vi "SolveSudoku_Labview.vi"() -> ()   [LabVIEW 2023]
uses:
  <vilib>/picture/picture.llb/imagedata.ctl
  <vilib>/Utility/error.llb/Error Cluster From Error Code.vi
  <vilib>/ErrorRing/Error Ring.xnode
panel:
  in  "oPENpdf":bool
  out "subset rect out":T1
  out "Analyse des pixels":bool[][](array[boolean])
  out "resulting number":string
  in  "appel du matlab":bool
  out "Gestion des erreurs":errorcluster
  out "standard error":string
  out "standard output":string
  out "Rectangle.bottom":i16
  out "Rectangle.right":i16
  out "image data":T2
  out "case analysée par le C":picture
  out "Sudoku en entrée":picture
  in  "path to JPEG file":path
  # "SUDOKU SOLVER  :  VEUILLIEZ INSERER UNE GRILLE DE SUDOKU NON RESOLUE DANS LE PORTE DOCUMENT JAUNE ET  LE PROGRAMME VOUS RENVERRA LE SUDOKU RESOLUE !!!\n                     (si vous rentrer une grille qui n'est pas solvable ou avec des dimensions qui ne sont pas normées, le programme vous renverra une erreur ou un warning)"
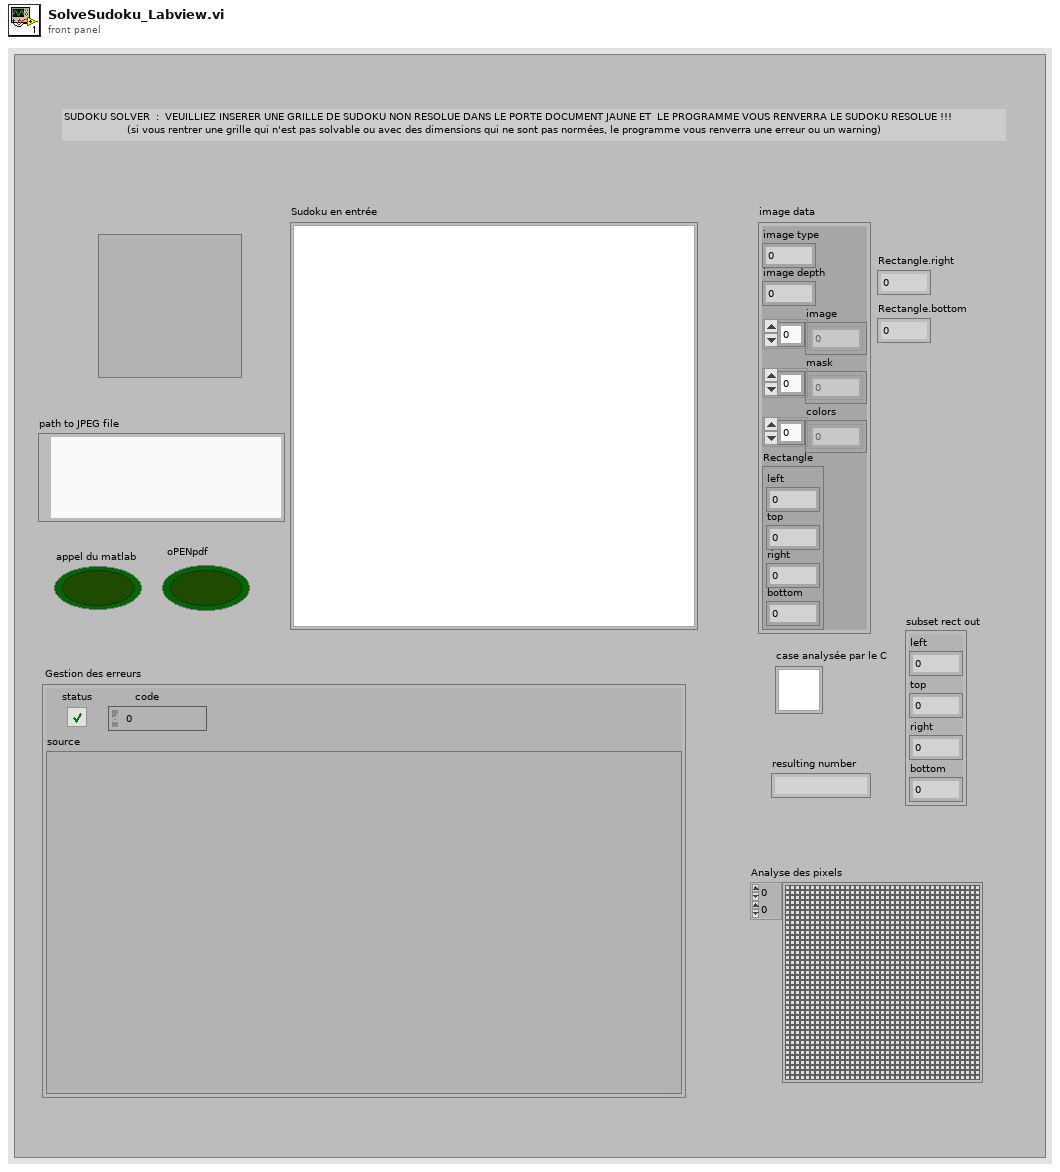
[diagram p1: front panel]
types:
  T1 = cluster{"left":i16, "top":i16, "right":i16, "bottom":i16}
  T2 = typedef "imagedata.ctl" = cluster{"image type":i32, "image depth":i32, "image":u8[], "mask":u8[], "colors":u32[], "Rectangle":cluster{"left":i16, "top":i16, "right":i16, "bottom":i16}}
  T3 = enum16{"open", "replace", "create", "open or create", "replace or create", "replace or create with confirmation"}
  T4 = enum16{"big-endian, network order", "native, host order", "little-endian"}
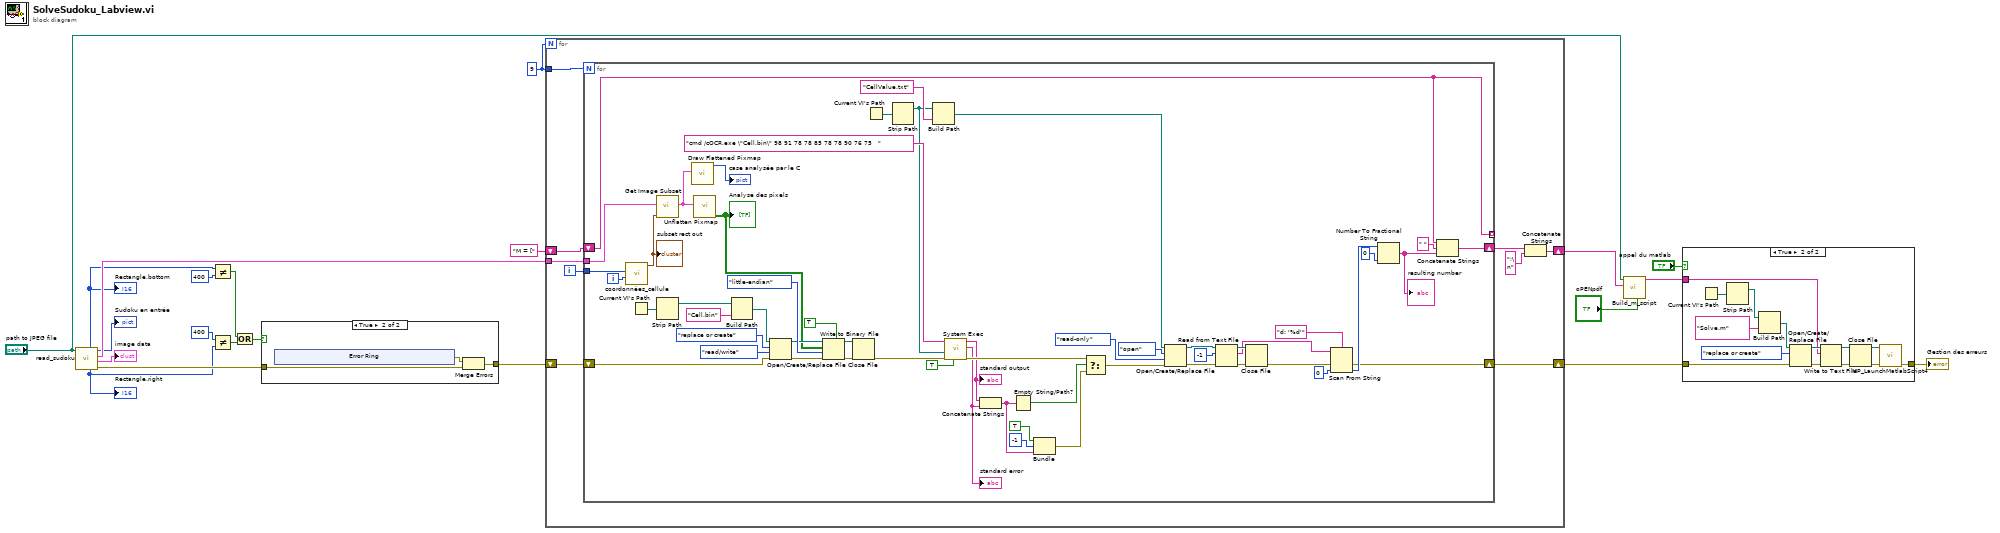
[diagram p0: block diagram]
diagram:
  w21 = 9
  n1 = call "read_sudoku.vi"("path to JPEG file"="path to JPEG file") -> ("gestion des erreurs"=w9:errorcluster, "image data"=→"image data":T2, "image data 2"=w12:T2, "new picture"=→"Sudoku en entrée":picture, "Rectangle.right"=w7:i16, "Rectangle.bottom"=w5:i16)  [unwired: 5 in]
  "Rectangle.right" <- w7
  "Rectangle.bottom" <- w5
  n2 = Not Equal?(x=w5, y=400) -> (x != y?=w3:bool)
  n3 = Not Equal?(x=400, y=w7) -> (x != y?=w2:bool)
  n4 = Or(x=w3, y=w2) -> (x .or. y?=w1:bool)
  n5 = case shown="True" w1 {
    tunnel: [w22 w23] -> w8
    tunnel: w9 -> [w22 w24]
    frame False {
    }
    frame True {
      n6 = xnode "Error Ring"() -> ("error out"=w25:errorcluster)
      n7 = Merge Errors(w25, w24) -> (w23:errorcluster)
    }
  }
  n8 = for {
    N: w21 -> [_]
    tunnel: w12 -> [w39]
    tunnel: w21 -> [w38]
    shift-right: [w34] -> w16
    shift-left: "M = [" ("String") -> [w33]
    shift-right: [w32] -> w19
    shift-left: w8 -> [w31]
    i -> [w37]
    n9 = for {
      N: w38 -> [_]
      tunnel: w39 -> [w91]
      tunnel: w37 -> [w53]
      shift-right: [w67] -> w36
      shift-left: w33 -> [w66]
      tunnel: [w66] -> _ mode=indexing
      shift-right: [w55] -> w32
      shift-left: w31 -> [w64]
      i -> [w52]
      n10 = call "coordonnées_cellule.vi"("Numeric"=w52, "Numeric 2"=w53) -> ("subset rect out"=w51:T1)  [unwired: 9 in]
      "subset rect out" <- w51
      n11 = Current VI's Path() -> (path=w78:path)
      n12 = call <vilib>:"Get Image Subset.vi"("subset rect"=w51, "image data"=w91) -> ("image subset"=w92:T2)  [unwired: 4 in, 1 out]
      n13 = Strip Path(path=w78) -> (stripped path=w90:path)  [unwired: 1 out]
      n14 = call <vilib>:"Draw Flattened Pixmap.vi"("image data"=w92) -> ("new picture"=→"case analysée par le C":picture)  [unwired: 8 in]
      n15 = call <vilib>:"Unflatten Pixmap.vi"("image data"=w92) -> ("1-bit pixmap"=w56:bool[][])  [unwired: 4 in, 6 out]
      "Analyse des pixels" <- w56
      n16 = Build Path(base path=w90, name or relative path="Cell.bin") -> (appended path=w79:path)
      n17 = Open/Create/Replace File(file path (use dialog)=w79, error in=w64, operation (0:open)=T3."replace or create", access (0:read/write)=enum16{"read/write", "read-only", "write-only"}."read/write") -> (refnum out=w57:refnum<file>, error out=w82:errorcluster)  [unwired: 2 in, 1 out]
      n18 = Write to Binary File(file (use dialog)=w57, data=w56, error in=w82, 5:TRUE ("prepend array or string size? (T)"), 9:T4."little-endian" ("byte order (0:big-endian, network order)")) -> (refnum out=w76:refnum<file>, error out=w77:errorcluster)  [unwired: 1 in, 1 out]
      n19 = Close File(refnum=w76, error in=w77) -> (error out=w75:errorcluster)  [unwired: 1 out]
      n20 = Current VI's Path() -> (path=w74:path)
      n21 = Strip Path(path=w74) -> (stripped path=w62:path)  [unwired: 1 out]
      n22 = Build Path(base path=w62, name or relative path="CellValue.txt") -> (appended path=w72:path)
      n23 = call <vilib>:"System Exec.vi"("run minimized? (F)"=TRUE, "error in (no error)"=w75, "working directory"=w62, "command line"="cmd /cOCR.exe \"Cell.bin\" 98 91 78 78 85 78 78 90 76 75   " ("standard input")) -> ("error out"=w47:errorcluster, "standard error"=w41:string, "standard output"=w42:string)  [unwired: 4 in, 1 out]
      "standard output" <- w42
      "standard error" <- w41
      n24 = Concatenate Strings(w42, w41) -> (w40:string)
      n25 = Empty String/Path?(string/path=w40) -> (empty?=w48:bool)
      n26 = Bundle("status"=TRUE, "code"=-1, w40) -> (w44:cluster{"status":bool, "code":i32, string})  [unwired: 1 in]
      n27 = Select(t=w47, s=w48, f=w44) -> (s? t:f=w43:errorcluster)
      n28 = Open/Create/Replace File(file path (use dialog)=w72, error in=w43, operation (0:open)=T3."open" ("operation (0:open) 2"), access (0:read/write)=enum16{"read/write", "read-only", "write-only"}."read-only") -> (refnum out=w87:refnum<file>, error out=w61:errorcluster)  [unwired: 2 in, 1 out]
      n29 = Read from Text File(file (use dialog)=w87, count=-1, error in=w61) -> (refnum out=w86:refnum<file>, text=w71:string, error out=w88:errorcluster)  [unwired: 1 in, 1 out]
      n30 = Close File(refnum=w86, error in=w88) -> (error out=w50:errorcluster)  [unwired: 1 out]
      n31 = Scan From String(format string="d: '%d'", input string=w71, error in=w50, default 1=i16 0 ("precision (6)")) -> (error out=w55:errorcluster, output 1=w70:i16)  [unwired: 1 in, 2 out]
      n32 = Number To Fractional String(number=w70, precision (6)=i16 0) -> (F-format string=w59:string)  [unwired: 2 in]
      "resulting number" <- w59
      n33 = Concatenate Strings(w66, " " ("string"), w59) -> (w67:string)
    }
    n34 = Concatenate Strings(w36, ";\n" ("string")) -> (w34:string)
  }
  n35 = call "Build_m_script.vi"("oPENpdf"="oPENpdf", "String in"=w16, "path to JPEG file"="path to JPEG file") -> ("String out"=w14:string)  [unwired: 8 in]
  n36 = case shown="True" "appel du matlab" {
    tunnel: w19 -> [w94 w97]
    tunnel: [w94 w96] -> w18
    tunnel: w14 -> [_ w95]
    frame False {
    }
    frame True {
      n37 = Current VI's Path() -> (path=w101:path)
      n38 = Strip Path(path=w101) -> (stripped path=w102:path)  [unwired: 1 out]
      n39 = Build Path(base path=w102, name or relative path="Solve.m" ("string")) -> (appended path=w100:path)
      n40 = Open/Create/Replace File(file path (use dialog)=w100, error in=w97, operation (0:open)=T3."replace or create") -> (refnum out=w108:refnum<file>, error out=w103:errorcluster)  [unwired: 3 in, 1 out]
      n41 = Write to Text File(file (use dialog)=w108, text=w95, error in=w103) -> (refnum out=w107:refnum<file>, error out=w104:errorcluster)  [unwired: 1 in, 1 out]
      n42 = Close File(refnum=w107, error in=w104) -> (path=w106:path, error out=w105:errorcluster)
      n43 = call "MP_LaunchMatlabScript4.vi"("error in (no error)"=w105, "matlab script path"=w106) -> ("error out"=w96:errorcluster)  [unwired: 4 in, 5 out]
    }
  }
  "Gestion des erreurs" <- w18
